vi "DefScrLog.vi"(7 "Operation":T1, 8 "error in (no error)":errorcluster, 11 "Def Settings":cluster{"DefScrPath":string, "LastOrder":string}) -> (0 "error out":errorcluster, 3 "Def Settings Out":cluster{"DefScrPath":string, "LastOrder":string})   [LabVIEW 2011]
uses:
  Strict Type Controls/Settings Operation.ctl
  <vilib>/Utility/config.llb/Read Key (String).vi
  <vilib>/Utility/config.llb/Write Key (String).vi
  <vilib>/Utility/config.llb/NI_LVConfig.lvlib
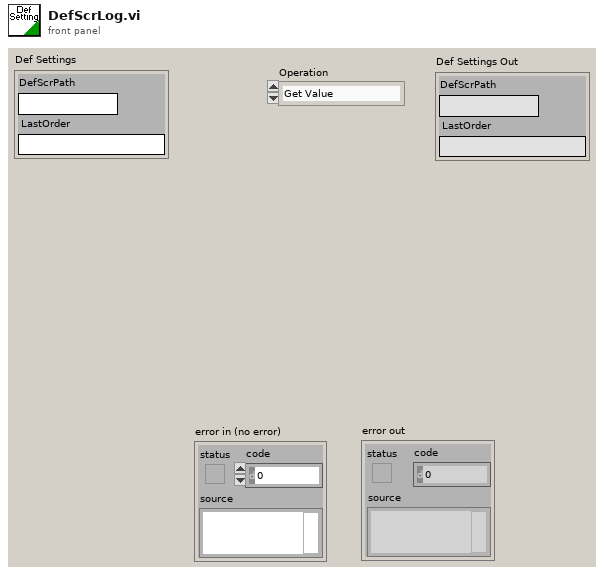
[diagram p1: front panel]
types:
  T1 = typedef "Settings Operation.ctl" = enum8{"Get Value", "Set Value", "Read File", "Write File", "Write Stored Value"}
  T2 = typedef "NI_LVConfig.lvlib/Config Data RefNum.ctl" = refnum<k1>
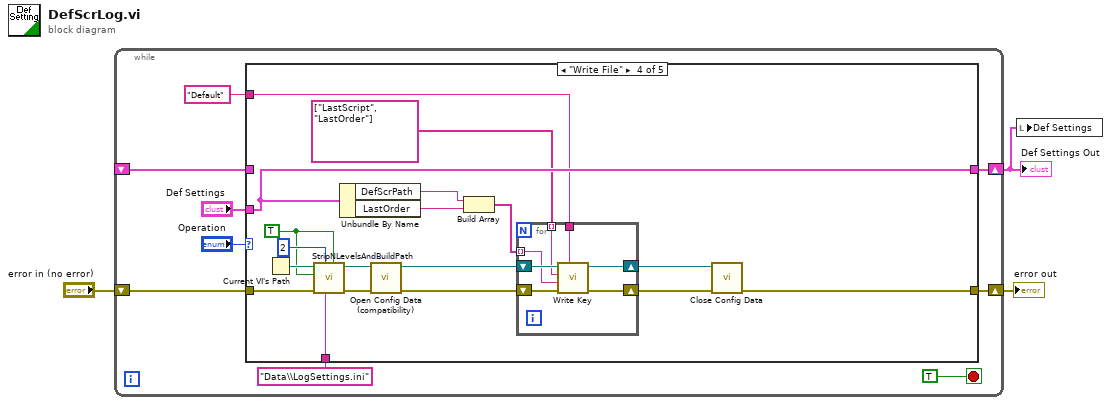
[diagram p0: block diagram]
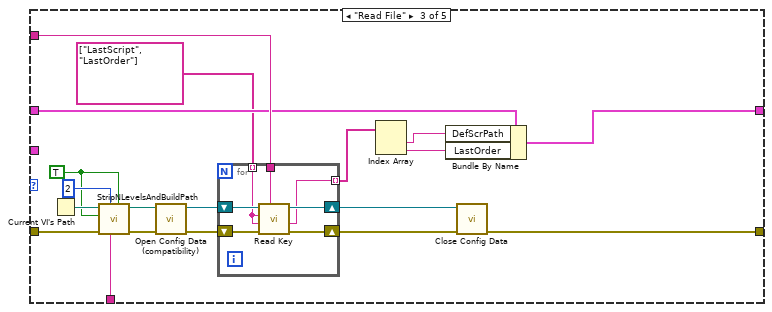
[diagram p4: hidden frame]
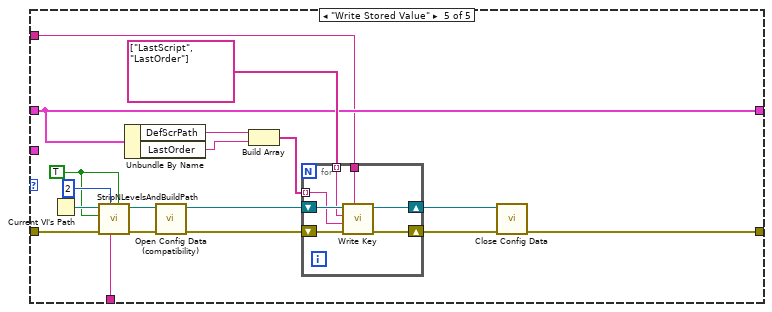
[diagram p5: hidden frame]
diagram:
  n1 = while {
    shift-right: [w11] -> w1
    shift-left: _ -> [w12]
    shift-right: [w8] -> w2
    shift-left: "error in (no error)" -> [w9]
    stop <- TRUE stop-if-true
    n2 = case shown="\"Write File\"" "Operation" {
      tunnel: w12 -> [w14 _ w24 _ w70]
      tunnel: [w14 w16 w23 w50 w70] -> w11
      tunnel: "Def Settings" -> [_ w16 _ w50 _]
      tunnel: w9 -> [w13 w15 w30 w59 w84]
      tunnel: [w13 w15 w20 w54 w79] -> w8
      tunnel: "Data\\LogSettings.ini" ("Build Path") -> [_ _ w29 w53 w78]
      tunnel: "Default" ("ScriptName") -> [_ _ w25 w45 w69]
      frame "Get Value" {
      }
      frame "Set Value" {
      }
      frame "Read File" {
        w33 = TRUE ("Is File?")
        n3 = Current VI's Path() -> (path=w35:path)
        n4 = call "StripNLevelsAndBuildPath.vi"("Create Folders"=w33, "Build Path"=w29, "Strip Levels"=2, "error in(no error)"=w30, "Is File"=w33, "Path In"=w35) -> ("error out"=w31:errorcluster, "Path Out"=w32:path)  [unwired: 4 out]
        n5 = call <vilib>:"Open Config Data (compatibility).vi"("error in (no error)"=w31, "configuration file path"=w32) -> ("error out"=w28:errorcluster, "refnum"=w27:T2)  [unwired: 7 in, 1 out]
        n6 = for {
          shift-right: [w40] -> w26
          shift-left: w27 -> [w42]
          shift-right: [w39] -> w21
          shift-left: w28 -> [w41]
          tunnel: string[] ["LastScript", "LastOrder"] ("appended array") -> [w38] mode=indexing
          tunnel: w25 -> [w37]
          tunnel: [w36] -> w22 mode=indexing
          n7 = call-poly <vilib>:"Read Key.vi"("section"=w37, "error in (no error)"=w41, "default value"=w38, "key"=w38, "refnum"=w42) -> ("error out"=w39:errorcluster, "value"=w36:string, "refnum out"=w40:T2)  [unwired: 1 in, 3 out]
        }
        n8 = Index Array(array=w22) -> (element #1=w17:string, element #2=w18:string)  [unwired: 2 in]
        n9 = Bundle By Name(cluster=w24, "DefScrPath"=w17, "LastOrder"=w18) -> (w23:cluster{"DefScrPath":string, "LastOrder":string})
        n10 = call <vilib>:"Close Config Data.vi"("error in (no error)"=w21, "refnum"=w26) -> ("error out"=w20:errorcluster)  [unwired: 1 in, 8 out]
      }
      frame "Write File" {
        w57 = TRUE ("Is File?")
        n11 = Current VI's Path() -> (path=w60:path)
        n12 = call "StripNLevelsAndBuildPath.vi"("Create Folders"=w57, "Build Path"=w53, "Strip Levels"=2, "error in(no error)"=w59, "Is File"=w57, "Path In"=w60) -> ("error out"=w55:errorcluster, "Path Out"=w56:path)  [unwired: 4 out]
        n13 = Unbundle By Name(w50) -> ("DefScrPath"=w43:string, "LastOrder"=w47:string)
        n14 = call <vilib>:"Open Config Data (compatibility).vi"("error in (no error)"=w55, "configuration file path"=w56) -> ("error out"=w51:errorcluster, "refnum"=w52:T2)  [unwired: 7 in, 1 out]
        n15 = Build Array(w43, w47) -> (w46:string[])
        n16 = for {
          tunnel: w46 -> [w63] mode=indexing
          shift-right: [w65] -> w49
          shift-left: w52 -> [w67]
          shift-right: [w64] -> w48
          shift-left: w51 -> [w66]
          tunnel: string[] ["LastScript", "LastOrder"] ("appended array") -> [w62] mode=indexing
          tunnel: w45 -> [w61]
          n17 = call-poly <vilib>:"Write Key.vi"("section"=w61, "error in (no error)"=w66, "value"=w63, "key"=w62, "refnum"=w67) -> ("error out"=w64:errorcluster, "refnum out"=w65:T2)  [unwired: 1 in, 4 out]
        }
        n18 = call <vilib>:"Close Config Data.vi"("error in (no error)"=w48, "refnum"=w49) -> ("error out"=w54:errorcluster)  [unwired: 1 in, 8 out]
      }
      frame "Write Stored Value" {
        w82 = TRUE ("Is File?")
        n19 = Current VI's Path() -> (path=w85:path)
        n20 = call "StripNLevelsAndBuildPath.vi"("Create Folders"=w82, "Build Path"=w78, "Strip Levels"=2, "error in(no error)"=w84, "Is File"=w82, "Path In"=w85) -> ("error out"=w80:errorcluster, "Path Out"=w81:path)  [unwired: 4 out]
        n21 = Unbundle By Name(w70) -> ("DefScrPath"=w68:string, "LastOrder"=w73:string)
        n22 = call <vilib>:"Open Config Data (compatibility).vi"("error in (no error)"=w80, "configuration file path"=w81) -> ("error out"=w76:errorcluster, "refnum"=w77:T2)  [unwired: 7 in, 1 out]
        n23 = Build Array(w68, w73) -> (w72:string[])
        n24 = for {
          tunnel: w72 -> [w88] mode=indexing
          shift-right: [w90] -> w75
          shift-left: w77 -> [w92]
          shift-right: [w89] -> w74
          shift-left: w76 -> [w91]
          tunnel: string[] ["LastScript", "LastOrder"] ("appended array") -> [w87] mode=indexing
          tunnel: w69 -> [w86]
          n25 = call-poly <vilib>:"Write Key.vi"("section"=w86, "error in (no error)"=w91, "value"=w88, "key"=w87, "refnum"=w92) -> ("error out"=w89:errorcluster, "refnum out"=w90:T2)  [unwired: 1 in, 4 out]
        }
        n26 = call <vilib>:"Close Config Data.vi"("error in (no error)"=w74, "refnum"=w75) -> ("error out"=w79:errorcluster)  [unwired: 1 in, 8 out]
      }
    }
  }
  "error out" <- w2
  "Def Settings Out" <- w1
  n27 = local write "Def Settings"(w1) -> ()
